vi "Output Enable Read Array.vi"(8 "error in":errorcluster, 11 "Power Supply In":refnum<class "Power Supply.lvclass">) -> (0 "error out":errorcluster, 2 "Output Enable ACT":bool[](array[boolean]), 3 "Power Supply Out":refnum<class "Power Supply.lvclass">)   [LabVIEW 2023, in "Power Supply.lvclass"]
uses:
  Power Supply.lvclass
  Power Supply.lvclass/Power Supply.ctl
  Low Level Capabilities/Output Enable/Output Enable.lvclass
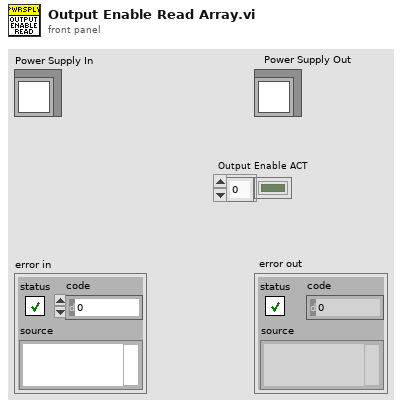
[diagram p1: front panel]
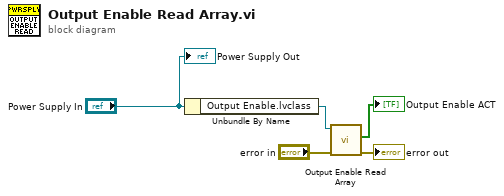
[diagram p0: block diagram]
diagram:
  n1 = Unbundle By Name("Power Supply In") -> ("Output Enable.lvclass"=w4:refnum<class "Output Enable.lvclass">)
  n2 = call-dynamic "Output Enable Read Array.vi"("error in"="error in", "Output Enable in"=w4) -> ("error out"=→"error out":errorcluster, "Output Enable ACT"=→"Output Enable ACT":bool[])  [unwired: 6 in, 2 out]
  "Power Supply Out" <- "Power Supply In"
